vi "Gyro Task.vi"(0 "GyroDevRef":T1, 1 "GyroDevRef 2":T1) -> ()   [LabVIEW 2011]
uses:
  <vilib>/Rock Robotics/WPI/Gyro/WPI_GyroDevRef.ctl
  <vilib>/Rock Robotics/SystemInterfaces/Typedef/FPGA_TypedefAnalogModule.ctl
  <vilib>/Rock Robotics/SystemInterfaces/AI/FPGA_AIChannel.ctl
  Robot Global Data.vi
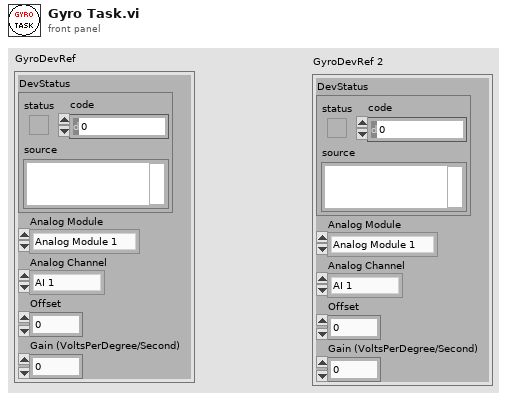
[diagram p1: front panel]
types:
  T1 = typedef "WPI_GyroDevRef.ctl" = cluster{"DevStatus":errorcluster, "Analog Module":T2, "Analog Channel":T3, "Offset":dbl, "Gain (VoltsPerDegree/Second)":dbl}
  T2 = typedef "FPGA_TypedefAnalogModule.ctl" = enum16{"Analog Module 1", "Analog Module 2"}
  T3 = typedef "FPGA_AIChannel.ctl" = enum8{"AI 1", "AI 2", "AI 3", "AI 4", "AI 5", "AI 6", "AI 7", "AI 8", "Invalid"}
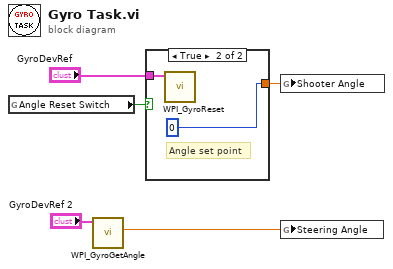
[diagram p0: block diagram]
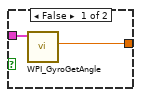
[diagram p2: hidden frame]
diagram:
  n1 = global read "Robot Global Data.vi" "Angle Reset Switch"() -> (w3:bool)
  n2 = call <vilib>:"WPI_GyroGetAngle.vi"("GyroDevRef"="GyroDevRef 2") -> ("Angle"=w4:dbl)  [unwired: 7 in, 3 out]
  n3 = case shown="True" w3 {
    tunnel: [w6 0] -> w2
    tunnel: "GyroDevRef" -> [w7 w8]
    frame False {
      n4 = call <vilib>:"WPI_GyroGetAngle.vi"("GyroDevRef"=w7) -> ("Angle"=w6:dbl)  [unwired: 7 in, 3 out]
    }
    frame True {
      # "Angle set point"
      n5 = call <vilib>:"WPI_GyroReset.vi"("GyroDevRef"=w8) -> ()  [unwired: 9 in, 2 out]
    }
  }
  n6 = global write "Robot Global Data.vi" "Shooter Angle"(w2) -> ()
  n7 = global write "Robot Global Data.vi" "Steering Angle"(w4) -> ()
